vi "Write AlicatSetup.vi"(8 "error in":errorcluster, 10 "AlicatSetup":T1, 11 "Alicat in":refnum<class "Alicat.lvclass">) -> (0 "error out":errorcluster, 3 "Alicat out":refnum<class "Alicat.lvclass">)   [LabVIEW 2014, in "Alicat.lvlib" / "Alicat.lvclass"]
doc: "Write the name, address, device full scale and the gas to the object."
uses:
  Alicat.lvclass
  Controls/CtlSetup.ctl
  Controls/Gas.ctl
  Alicat.lvclass/Alicat.ctl
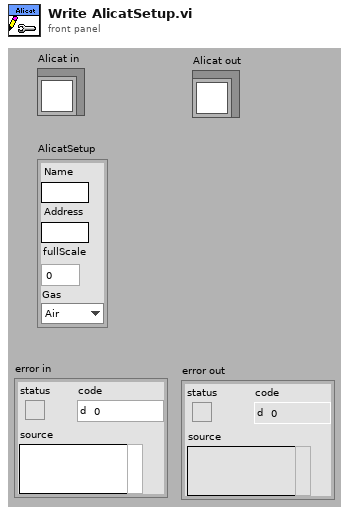
[diagram p1: front panel]
types:
  T1 = typedef "Alicat.lvlib/Alicat.lvclass/CtlSetup.ctl" = cluster{"Name":string, "Address":string, "fullScale":dbl, "Gas":T2}
  T2 = typedef "Alicat.lvlib/Alicat.lvclass/Gas.ctl" = enum16{"Air", "Ar", "CH4", "CO", "CO2", "C2H6", "H2", "He", "N2", "NO", "Ne", "O2", "C3H8", "n-C4H10", "C2H2", "C2H4", "i-C2H10", "Kr", "Xe"}
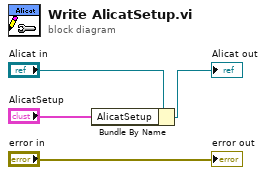
[diagram p0: block diagram]
diagram:
  n1 = Bundle By Name(cluster="Alicat in", "AlicatSetup"="AlicatSetup") -> (→"Alicat out":refnum<class "Alicat.lvclass">)
  "error out" <- "error in"
